vi "Autonomous Independent.vi"() -> ()   [LabVIEW 2015]
doc: "This VI is called when autonomous begins, and will automatically be terminated when autonomous ends. You can carry out timed or sensor driven robot movement independently without needing to return to the caller."
uses:
  <vilib>/Rock Robotics/Network Tables/NT Read Number.vi
  Robot Global Data.vi
  <vilib>/addons/control/pid/NI_PID_pid.lvlib
  <vilib>/addons/control/pid/pid.llb/PID (DBL).vi
panel:
  out "camera":dbl
  out "output":dbl format="%.2f"
  in  "output range":cluster{"output high":dbl, "output low":dbl}={"output high"=100.0, "output low"=-100.0} {"output low" format="%.2f"; "output high" format="%.2f"}
  in  "PID gains":T1={"proportional gain (Kc)"=1.0, "integral time (Ti, min)"=0.01, "derivative time (Td, min)"=0.0} {"derivative time (Td, min)" format="%.3f"; "integral time (Ti, min)" format="%.3f"; "proportional gain (Kc)" format="%.3f"}
  out "centerHoriz":dbl
  out "Starting Position":dbl
  out "Defense to Cross":dbl
  # "0 - Low Bar (Far Left)\n4 - Far Right"
  # "0 - Low Bar\n1 - Porticullis\n2 - Shovel the Fries\n3 - Moat\n4 - Ramparts\n5 - Rough Terrain\n6 - Rock Wall"
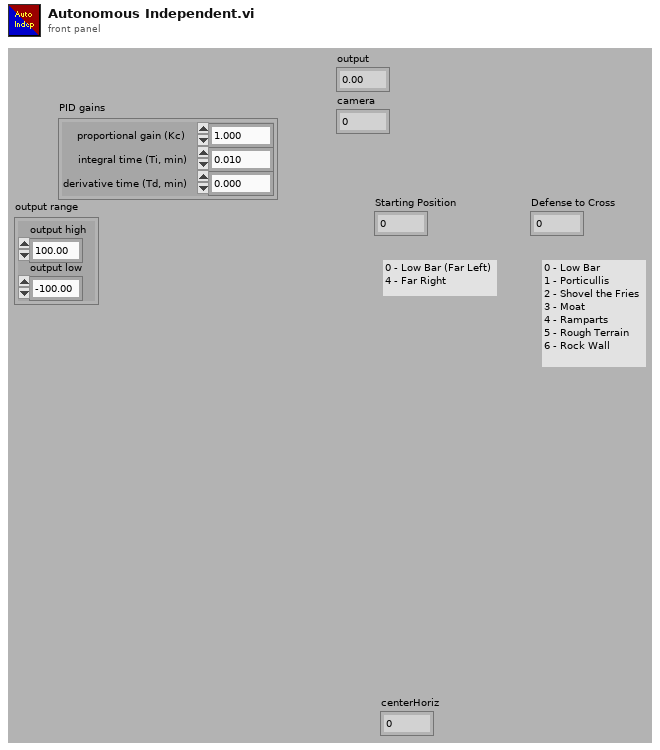
[diagram p1: front panel]
types:
  T1 = cluster{"proportional gain (Kc)":dbl, "integral time (Ti, min)":dbl, "derivative time (Td, min)":dbl}
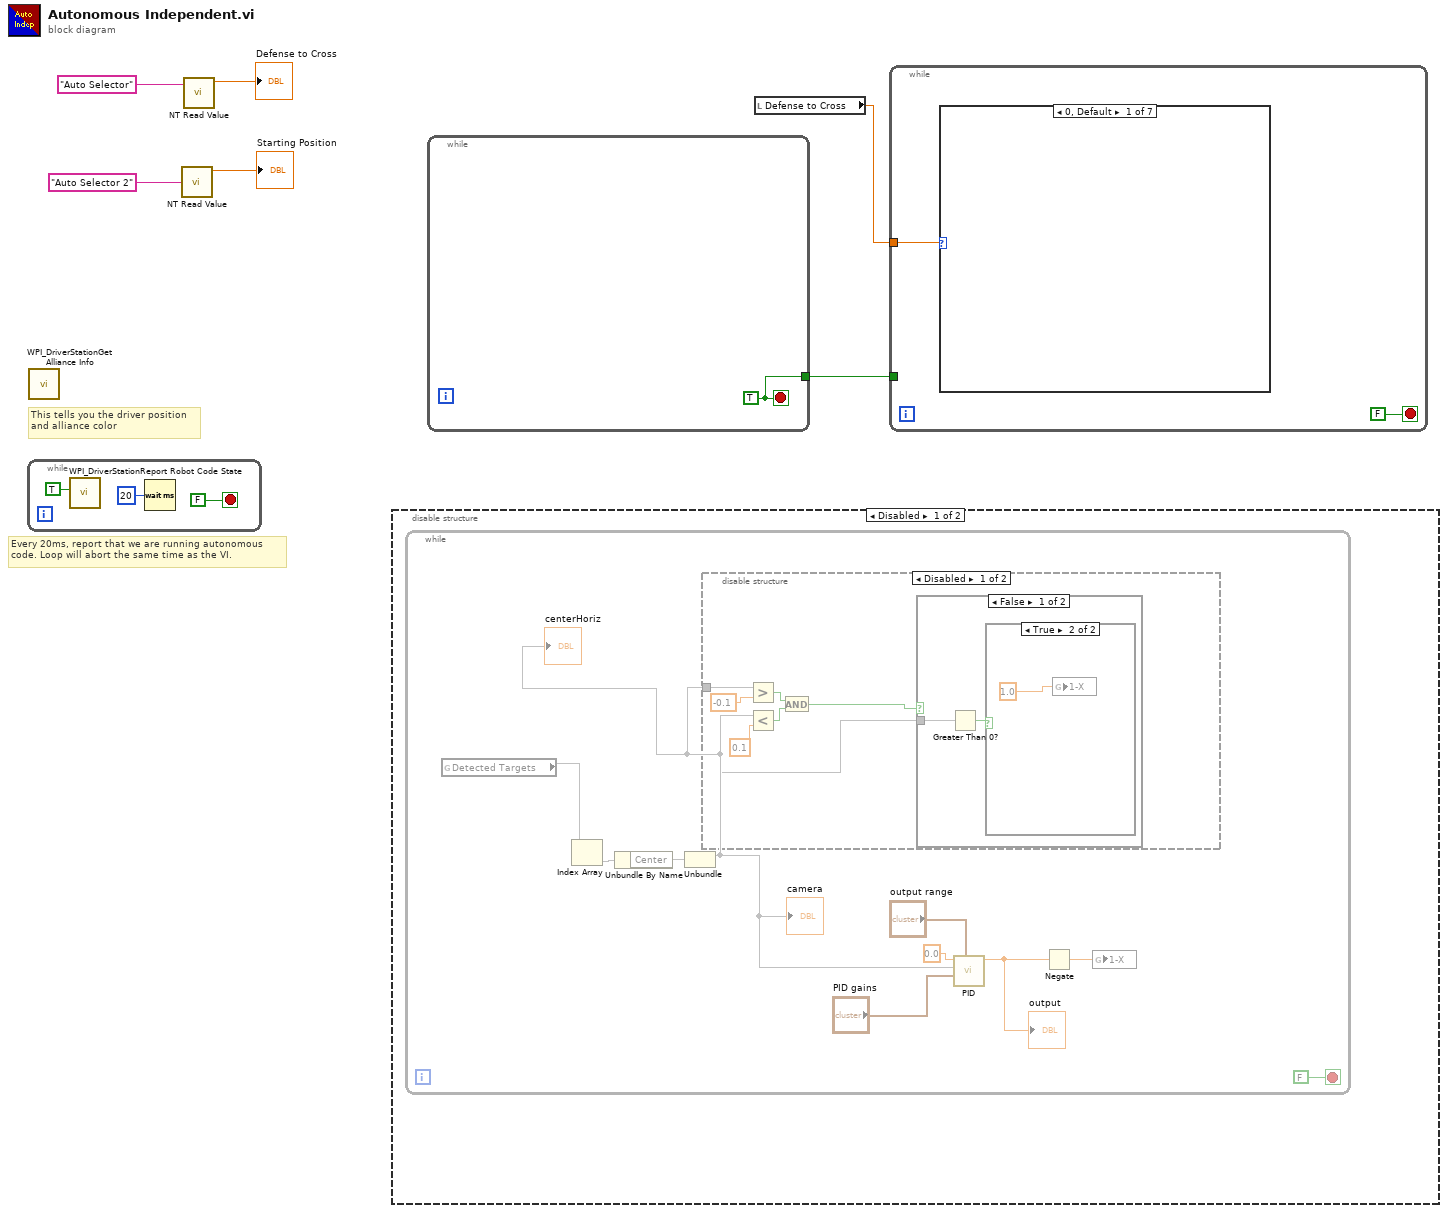
[diagram p0: block diagram]
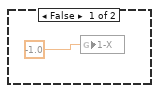
[diagram p2: hidden frame]
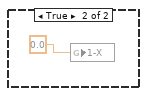
[diagram p3: hidden frame]
diagram:
  # "Every 20ms, report that we are running autonomous\ncode. Loop will abort the same time as the VI."
  # "This tells you the driver position\nand alliance color"
  n1 = while {
    stop <- FALSE stop-if-true
    n2 = call <vilib>:"WPI_DriverStationReport Robot Code State.vi"("Autonomous"=TRUE) -> ()  [unwired: 10 in, 1 out]
    n3 = Wait (ms)(milliseconds to wait=u32 20) -> ()  [unwired: 1 out]
  }
  n4 = call <vilib>:"WPI_DriverStationGet Alliance Info.vi"() -> ()  [unwired: 12 out]
  n5 = call-poly <vilib>:"NT Read Value.vi"("Name"="Auto Selector 2") -> ("Numeric"=→"Starting Position":dbl)  [unwired: 9 in, 1 out]
  n6 = call-poly <vilib>:"NT Read Value.vi"("Name"="Auto Selector") -> ("Numeric"=→"Defense to Cross":dbl)  [unwired: 9 in, 1 out]
  n7 = disable-structure shown="Disabled" {
    frame Disabled {
      n8 = while {
        stop <- FALSE stop-if-true
        n9 = global read "Robot Global Data.vi" "Detected Targets"() -> (w19)
        n10 = Index Array(array=w19) -> (element=w18)  [unwired: 1 in]
        n11 = Unbundle By Name(w18) -> ("Center"=w17)
        n12 = Unbundle(w17) -> (w14)  [unwired: 1 out]
        "centerHoriz" <- w14
        "camera" <- w14
        n13 = disable-structure shown="Disabled" {
          disable-tunnel: w14 -> [w20 _]
          frame Disabled {
            n14 = Greater?(x=w20, y=-0.1) -> (0:w25:bool)
            n15 = Less?(x=w20, y=0.1) -> (x < y?=w24:bool)
            n16 = And(x=w25, y=w24) -> (x .and. y?=w21:bool)
            n17 = case shown="False" w21 {
              tunnel: w20 -> [w26 _]
              frame False {
                n18 = Greater Than 0?(x=w26) -> (x > 0?=w27:bool)
                n19 = case shown="True" w27 {
                  frame False {
                    n20 = global write "Robot Global Data.vi" "1-X"(-1.0 ("1-X")) -> ()
                  }
                  frame True {
                    n21 = global write "Robot Global Data.vi" "1-X"(1.0 ("1-X")) -> ()
                  }
                }
              }
              frame True {
                n22 = global write "Robot Global Data.vi" "1-X"(0.0 ("1-X")) -> ()
              }
            }
          }
          frame Enabled {
          }
        }
        n23 = call-poly <vilib>:"PID.vi"("output range"="output range", "PID gains"="PID gains", "process variable"=w14, "setpoint"=0.0) -> ("output"=w10:dbl)  [unwired: 6 in, 1 out]
        "output" <- w10
        n24 = Negate(x=w10) -> (-x=w11:dbl)
        n25 = global write "Robot Global Data.vi" "1-X"(w11) -> ()
      }
    }
    frame Enabled {
    }
  }
  n26 = while {
    tunnel: [w31] -> w1
    stop <- w31 stop-if-true
    w31 = TRUE
  }
  n27 = local read "Defense to Cross"() -> (w2:dbl)
  n28 = while {
    tunnel: w2 -> [w33]
    tunnel: w1 -> [_]
    stop <- FALSE stop-if-true
    n29 = case shown="0, Default" w33 {
      frame 0, Default {
      }
      frame 1 {
      }
      frame 2 {
      }
      frame 3 {
      }
      frame 4 {
      }
      frame 5 {
      }
      frame 6 {
      }
    }
  }
